vi "Test Map Range not in map.vi"(8 "error in (no error)":errorcluster, 11 "Test Case In":refnum<class "Revisit Test.lvclass">) -> (0 "error out":errorcluster, 3 "Test Case Out":refnum<class "Revisit Test.lvclass">)   [LabVIEW 2020, in "Revisit Test.lvclass"]
uses:
  Revisit Test.lvclass
  Revisit Test.lvclass/Revisit Test.ctl
  4993e8ee-a06a-463a-9684-69129f64d5ce.vi
  Range Map/Range Map.lvclass
  Range/Range.lvclass
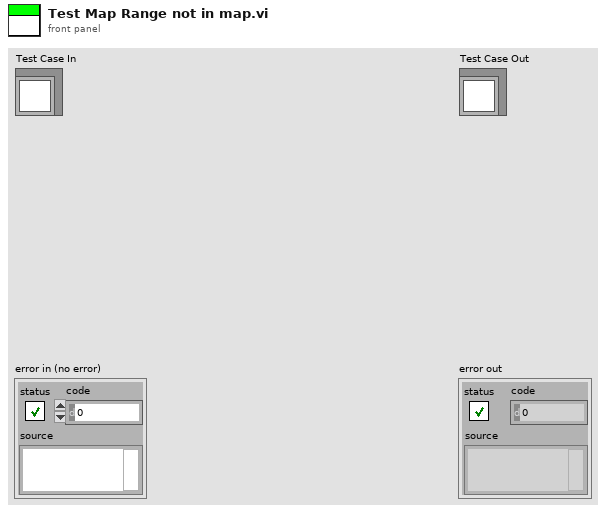
[diagram p1: front panel]
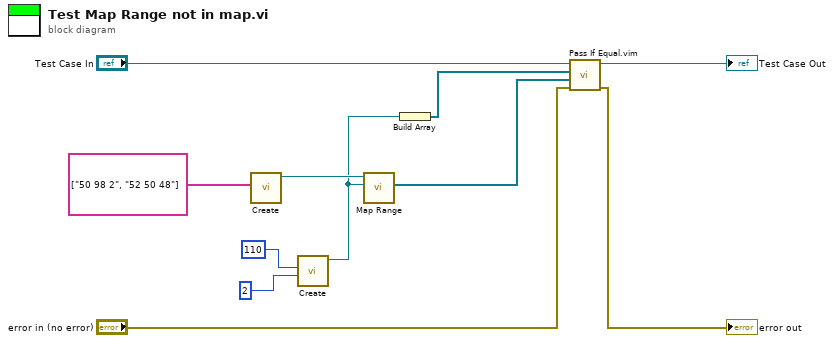
[diagram p0: block diagram]
diagram:
  n1 = call "Create.vi"("Input"=string[] ["50 98 2", "52 50 48"] ("string array")) -> ("Range Map"=w5:refnum<class "Range Map.lvclass">)  [unwired: 9 in, 1 out]
  n2 = call "Create.vi"("Length"=u64 2, "From"=u64 110) -> ("Range"=w1:refnum<class "Range.lvclass">)  [unwired: 8 in, 1 out]
  n3 = call "Map Range.vi"("Range"=w1, "Range Map in"=w5) -> ("Ranges"=w3:refnum<class "Range.lvclass">[])  [unwired: 7 in, 2 out]
  n4 = Build Array(w1) -> (w4:refnum<class "Range.lvclass">[])
  n5 = call "Pass If Equal.vim"("error in (no error)"="error in (no error)", "Actual"=w3, "Expected"=w4, "LUnit Test Case In"="Test Case In") -> ("error out"=→"error out":errorcluster, "LUnit Test Case Out"=→"Test Case Out":refnum<class "Revisit Test.lvclass">)  [unwired: 6 in]
